vi "new dp ro.vi"() -> ()   [LabVIEW 2013]
doc: "Use this template to build a standard state machine design pattern. Each state executes code and determines which state to transition to. Contrast this design pattern with the User Interface Event Handler pattern, in which code executes in response to user actions. Contrast this design pattern also with the Queued Message Handler pattern, in which each message handling code can queue zero or more new messages.\nNote: This template does not contain the most recent programming guidelines recommended by National Instruments. For a complete, project-based implementation of the Standard State Machine pattern, use the Create Project dialog box instead of this template."
uses:
  StateMachineStates 2.ctl
panel:
  out "Water":string
  in  "on/off":bool
  in  "Dispense":bool
  out "Indicator":cluster{"Red":bool, "Yellow":bool, "Green":bool}
  # "Red- Receive Water\nYellow-Process Water\nGreen- Ready to dispense\nwater"
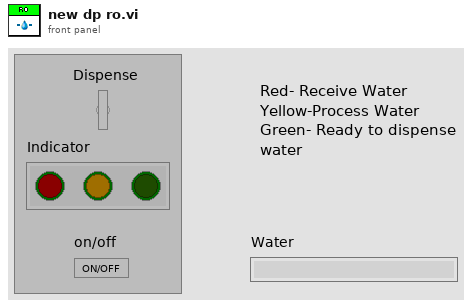
[diagram p1: front panel]
types:
  T1 = typedef "StateMachineStates 2.ctl" = enum16{"Initialize", "Main", "Start", "Receive Value", "Process value", "Signal Water Ready", "Dispense Water", "Stop"}
  T2 = enum8{"Enabled", "Disabled", "Disabled and Grayed Out"}
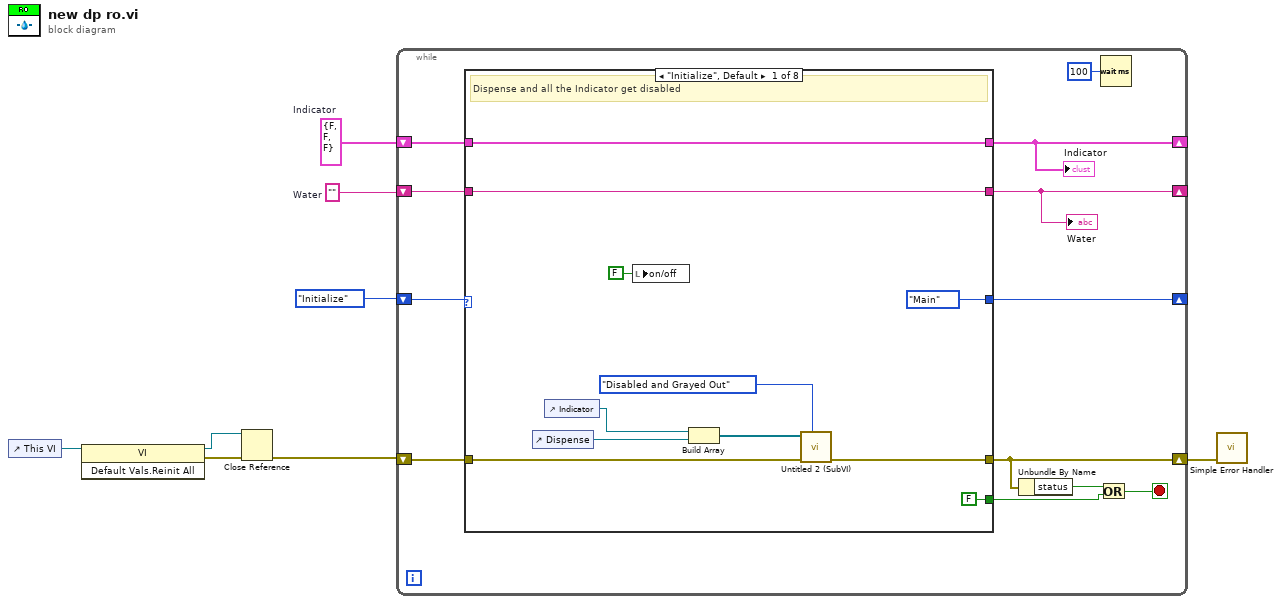
[diagram p0: block diagram]
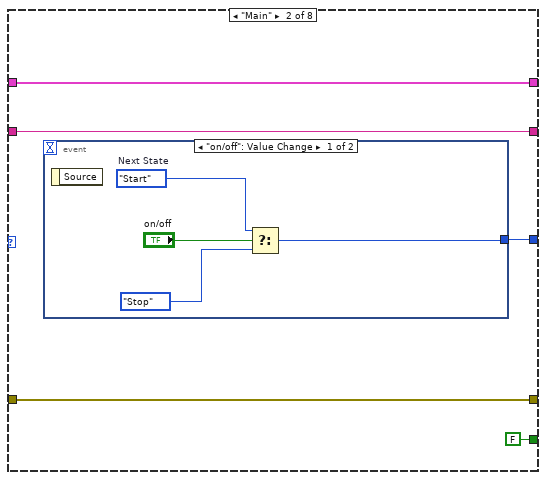
[diagram p2: hidden frame]
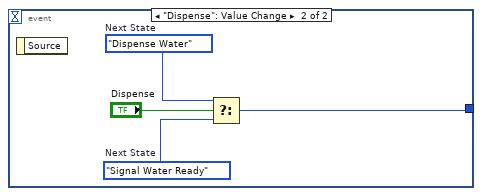
[diagram p3: hidden frame]
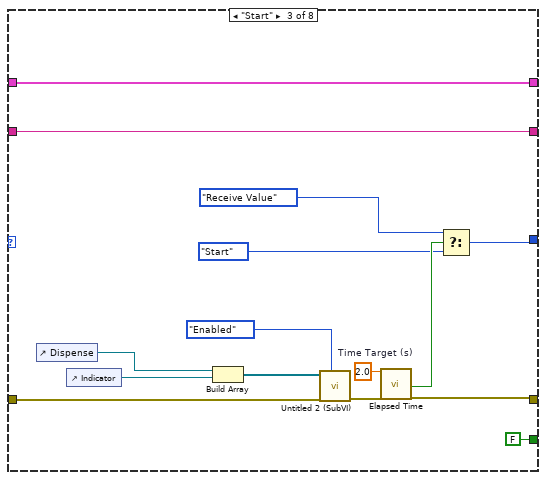
[diagram p4: hidden frame]
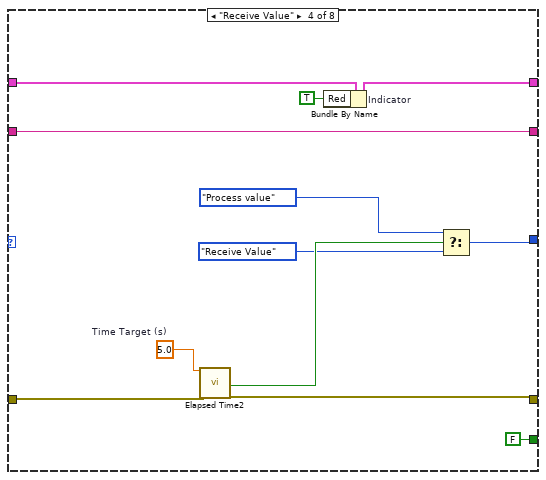
[diagram p5: hidden frame]
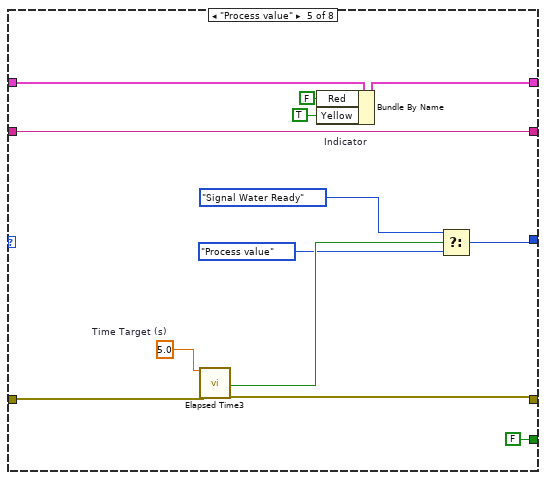
[diagram p6: hidden frame]
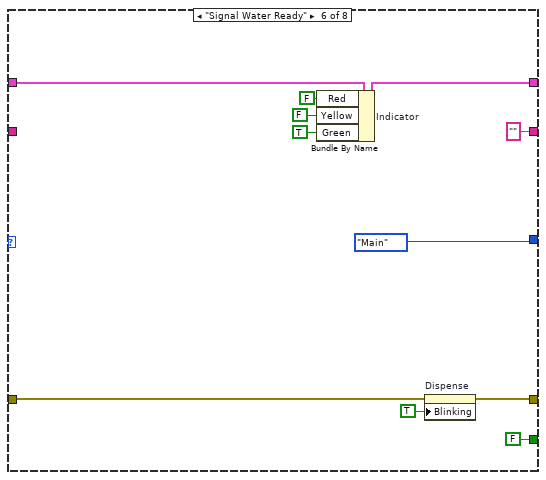
[diagram p7: hidden frame]
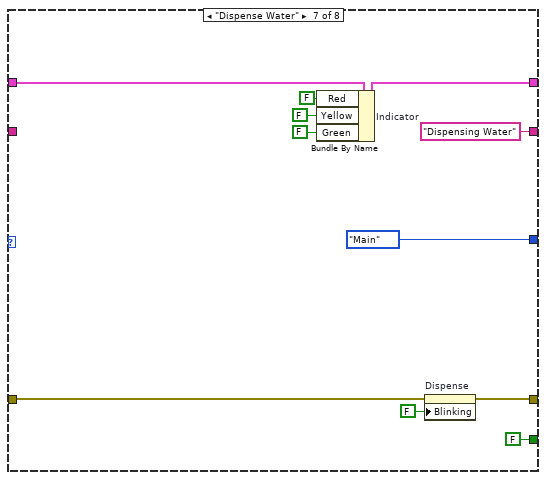
[diagram p8: hidden frame]
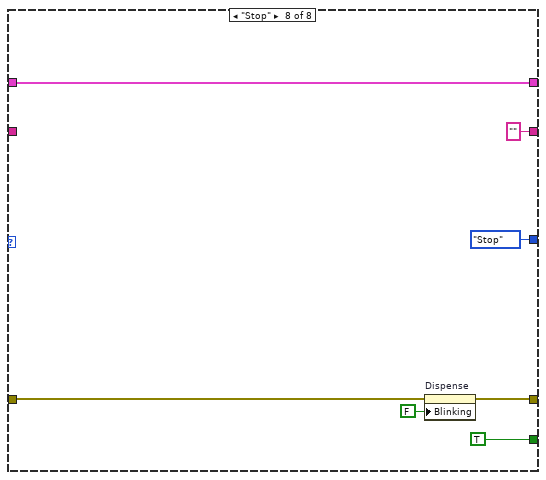
[diagram p9: hidden frame]
diagram:
  w6 = ""  # Water
  w7 = cluster{"Red":bool, "Yellow":bool, "Green":bool} {"Red"=FALSE, "Yellow"=FALSE, "Green"=FALSE}  # Indicator
  n1 = control-ref of="This VI"() -> (w4:refnum<vi>)
  n2 = invoke class="VI" method="Default Vals.Reinit All"(reference=w4) -> (reference out=w1:refnum<vi>, error out=w2:errorcluster)  [unwired: 2 in, 1 out]
  n3 = Close Reference(reference=w1, error in (no error)=w2) -> (error out=w3:errorcluster)
  n4 = while {
    shift-right: [w19] -> _
    shift-left: StateMachineStates_2."Initialize" ("Beginning State") -> [w20]
    shift-right: [w16] -> _
    shift-left: w7 -> [w17]
    shift-right: [w14] -> w5
    shift-left: w3 -> [w15]
    shift-right: [w9] -> _
    shift-left: w6 -> [w10]
    stop <- w11 stop-if-true
    n5 = case shown="\"Initialize\", Default" w20 {
      tunnel: [StateMachineStates_2."Main" ("Next State") w36 w52 w66 w79 StateMachineStates_2."Main" ("Beginning State") StateMachineStates_2."Main" ("Beginning State") StateMachineStates_2."Stop" ("Beginning State")] -> w19
      tunnel: [w26 w34 w53 w64 w77 w94 w105 w109] -> w16
      tunnel: w17 -> [w26 w34 w53 w67 w80 w95 w106 w109]
      tunnel: w15 -> [w28 w33 w51 w62 w75 w88 w99 w111]
      tunnel: [w27 w33 w49 w65 w78 w90 w101 w113] -> w14
      tunnel: [FALSE FALSE FALSE FALSE FALSE FALSE FALSE TRUE] -> w12
      tunnel: w10 -> [w24 w35 w47 w61 w73 _ _ _]
      tunnel: [w24 w35 w47 w61 w73 "" ("Water") "Dispensing Water" ("Water") "" ("Water")] -> w9
      frame "Initialize", Default {
        # "Dispense and all the Indicator get disabled"
        n6 = control-ref of="Dispense"() -> (w22:refnum<vi>)
        n7 = control-ref of="Indicator"() -> (w30:refnum<vi>)
        n8 = local write "on/off"(FALSE ("on/off")) -> ()
        n9 = Build Array(w30, w22) -> (w29:refnum<vi>[])
        n10 = call "Untitled 2 (SubVI).vi"("Disabled"=T2."Disabled and Grayed Out", "error in (no error)"=w28, "Array"=w29) -> ("error out"=w27:errorcluster)  [unwired: 8 in]
      }
      frame "Main" {
        n11 = event shown="[0] \"on/off\": Value Change" {
          selector: _ -> [_ _]
          dyn-events: _ -> [_ _]
          timeout: _ -> [_ _]
          tunnel: [w37 w41] -> w36
          event "on/off": Value Change {
            w39 = StateMachineStates_2."Start"  # Next State
            n12 = event-data() -> ()  [unwired: 1 in, 1 out]
            n13 = Select(t=w39, s="on/off", f=StateMachineStates_2."Stop") -> (s? t:f=w37:T1)
          }
          event "Dispense": Value Change {
            w43 = StateMachineStates_2."Signal Water Ready"  # Next State
            w42 = StateMachineStates_2."Dispense Water"  # Next State
            n14 = event-data() -> ()  [unwired: 1 in, 1 out]
            n15 = Select(t=w42, s="Dispense", f=w43) -> (s? t:f=w41:T1)
          }
        }
      }
      frame "Start" {
        w58 = 2.0  # Time Target (s)
        n16 = control-ref of="Dispense"() -> (w45:refnum<vi>)
        n17 = control-ref of="Indicator"() -> (w55:refnum<vi>)
        n18 = Build Array(w45, w55) -> (w50:refnum<vi>[])
        n19 = call "Untitled 2 (SubVI).vi"("Disabled"=T2."Enabled", "error in (no error)"=w51, "Array"=w50) -> ("error out"=w59:errorcluster)  [unwired: 8 in]
        n20 = call "Elapsed Time"("Time Target (s)"=w58, "error in (no error)"=w59) -> ("Time has Elapsed"=w57:bool, "error out"=w49:errorcluster)  [unwired: 10 in, 6 out]
        n21 = Select(t=StateMachineStates_2."Receive Value" ("Beginning State"), s=w57, f=StateMachineStates_2."Start" ("Beginning State")) -> (s? t:f=w52:T1)
      }
      frame "Receive Value" {
        w71 = 5.0  # Time Target (s)
        n22 = call "Elapsed Time2"("Time Target (s)"=w71, "error in (no error)"=w62) -> ("Time has Elapsed"=w70:bool, "error out"=w65:errorcluster)  [unwired: 10 in, 6 out]
        n23 = Bundle By Name "Indicator"(cluster=w67, "Red"=TRUE) -> (w64:cluster{"Red":bool, "Yellow":bool, "Green":bool})
        n24 = Select(t=StateMachineStates_2."Process value" ("Beginning State"), s=w70, f=StateMachineStates_2."Receive Value" ("Beginning State")) -> (s? t:f=w66:T1)
      }
      frame "Process value" {
        w84 = 5.0  # Time Target (s)
        n25 = call "Elapsed Time3"("Time Target (s)"=w84, "error in (no error)"=w75) -> ("Time has Elapsed"=w83:bool, "error out"=w78:errorcluster)  [unwired: 10 in, 6 out]
        n26 = Bundle By Name "Indicator"(cluster=w80, "Red"=FALSE, "Yellow"=TRUE) -> (w77:cluster{"Red":bool, "Yellow":bool, "Green":bool})
        n27 = Select(t=StateMachineStates_2."Signal Water Ready" ("Beginning State"), s=w83, f=StateMachineStates_2."Process value" ("Beginning State")) -> (s? t:f=w79:T1)
      }
      frame "Signal Water Ready" {
        n28 = Bundle By Name "Indicator"(cluster=w95, "Red"=FALSE, "Yellow"=FALSE, "Green"=TRUE) -> (w94:cluster{"Red":bool, "Yellow":bool, "Green":bool})
        n29 = property on="Dispense" class="Bool (strict)"(error in=w88, "Blinking"=TRUE) -> (error out=w90:errorcluster)  [unwired: 1 in, 1 out]
      }
      frame "Dispense Water" {
        n30 = Bundle By Name "Indicator"(cluster=w106, "Red"=FALSE, "Yellow"=FALSE, "Green"=FALSE) -> (w105:cluster{"Red":bool, "Yellow":bool, "Green":bool})
        n31 = property on="Dispense" class="Bool (strict)"(error in=w99, "Blinking"=FALSE) -> (error out=w101:errorcluster)  [unwired: 1 in, 1 out]
      }
      frame "Stop" {
        n32 = property on="Dispense" class="Bool (strict)"(error in=w111, "Blinking"=FALSE) -> (error out=w113:errorcluster)  [unwired: 1 in, 1 out]
      }
    }
    "Indicator" <- w16
    "Water" <- w9
    n33 = Unbundle By Name(w14) -> ("status"=w13:bool)
    n34 = Or(x=w13, y=w12) -> (x .or. y?=w11:bool)
    n35 = Wait (ms)(milliseconds to wait=u32 100) -> ()  [unwired: 1 out]
  }
  n36 = call <vilib>:"Simple Error Handler.vi"("error in (no error)"=w5) -> ()  [unwired: 4 in, 5 out]
